vi "estructura basica video tiempo real reconocimiento patrones extraccion de imagen 2.0.vi"() -> ()   [LabVIEW 2024]
uses:
  <vilib>/userDefined/High Color/IMAQdx.ctl
  <vilib>/Python/Open Anaconda Python Session.vi
  <vilib>/vision/driver/NI_Vision_Acquisition_Software.lvlib
  <vilib>/vision/NI_Vision_Development_Module.lvlib
panel:
  in  "Stop All":bool
  in  "Refresh Button":bool
  out "Elapsed Time (s)":dbl
  in  "Array 2":i32[][](array[numeric])
  out "Salida":i32[](array[numeric])
  out "error out":errorcluster
  out "Suma":dbl
  out "min value":u8
  out "max value":u8
  out "Promedio":dbl
  out "IMAGEN PROCESADA":T1(plugin-control)
  in  "Session In":T2="cam1"
  in  "Next":bool
  in  "Parameters (Pattern Matching 1)":T3={"Number of Matches Requested"=3, "Minimum Match Score"=800.0, "Angle Ranges"=[{"Start Angle"=-62.0, "End Angle"=54.0}]}
  out "Image 2":T1(plugin-control)
  out "Image 3":T1(plugin-control)
  in  "Template File Path (Pattern Matching 1)":path=path "C:/Users/cseba/OneDrive/Escritorio/C4.png"
  out "Image 4":T1(plugin-control)
  out "ROI":T4={"Global Rectangle"=[34, 35, 224, 222], "Contours"=[{"Contour Type"=0, "ROI Type"=3, "Points"=[34, 35, 224, 222]}]}
  # "1ER CUADRANTE"
  # "262, 306, 382, 428"
  # "2D0 CUADRANTE"
  # "448, 312, 562, 426"
  # "3ER CUADRANTE"
  # "628, 312, 746, 428"
  # "4TO CUADRANTE"
  # "814, 312, 924, 428"
  # "5TO CUADRANTE"
  # "996, 312, 1110, 424"
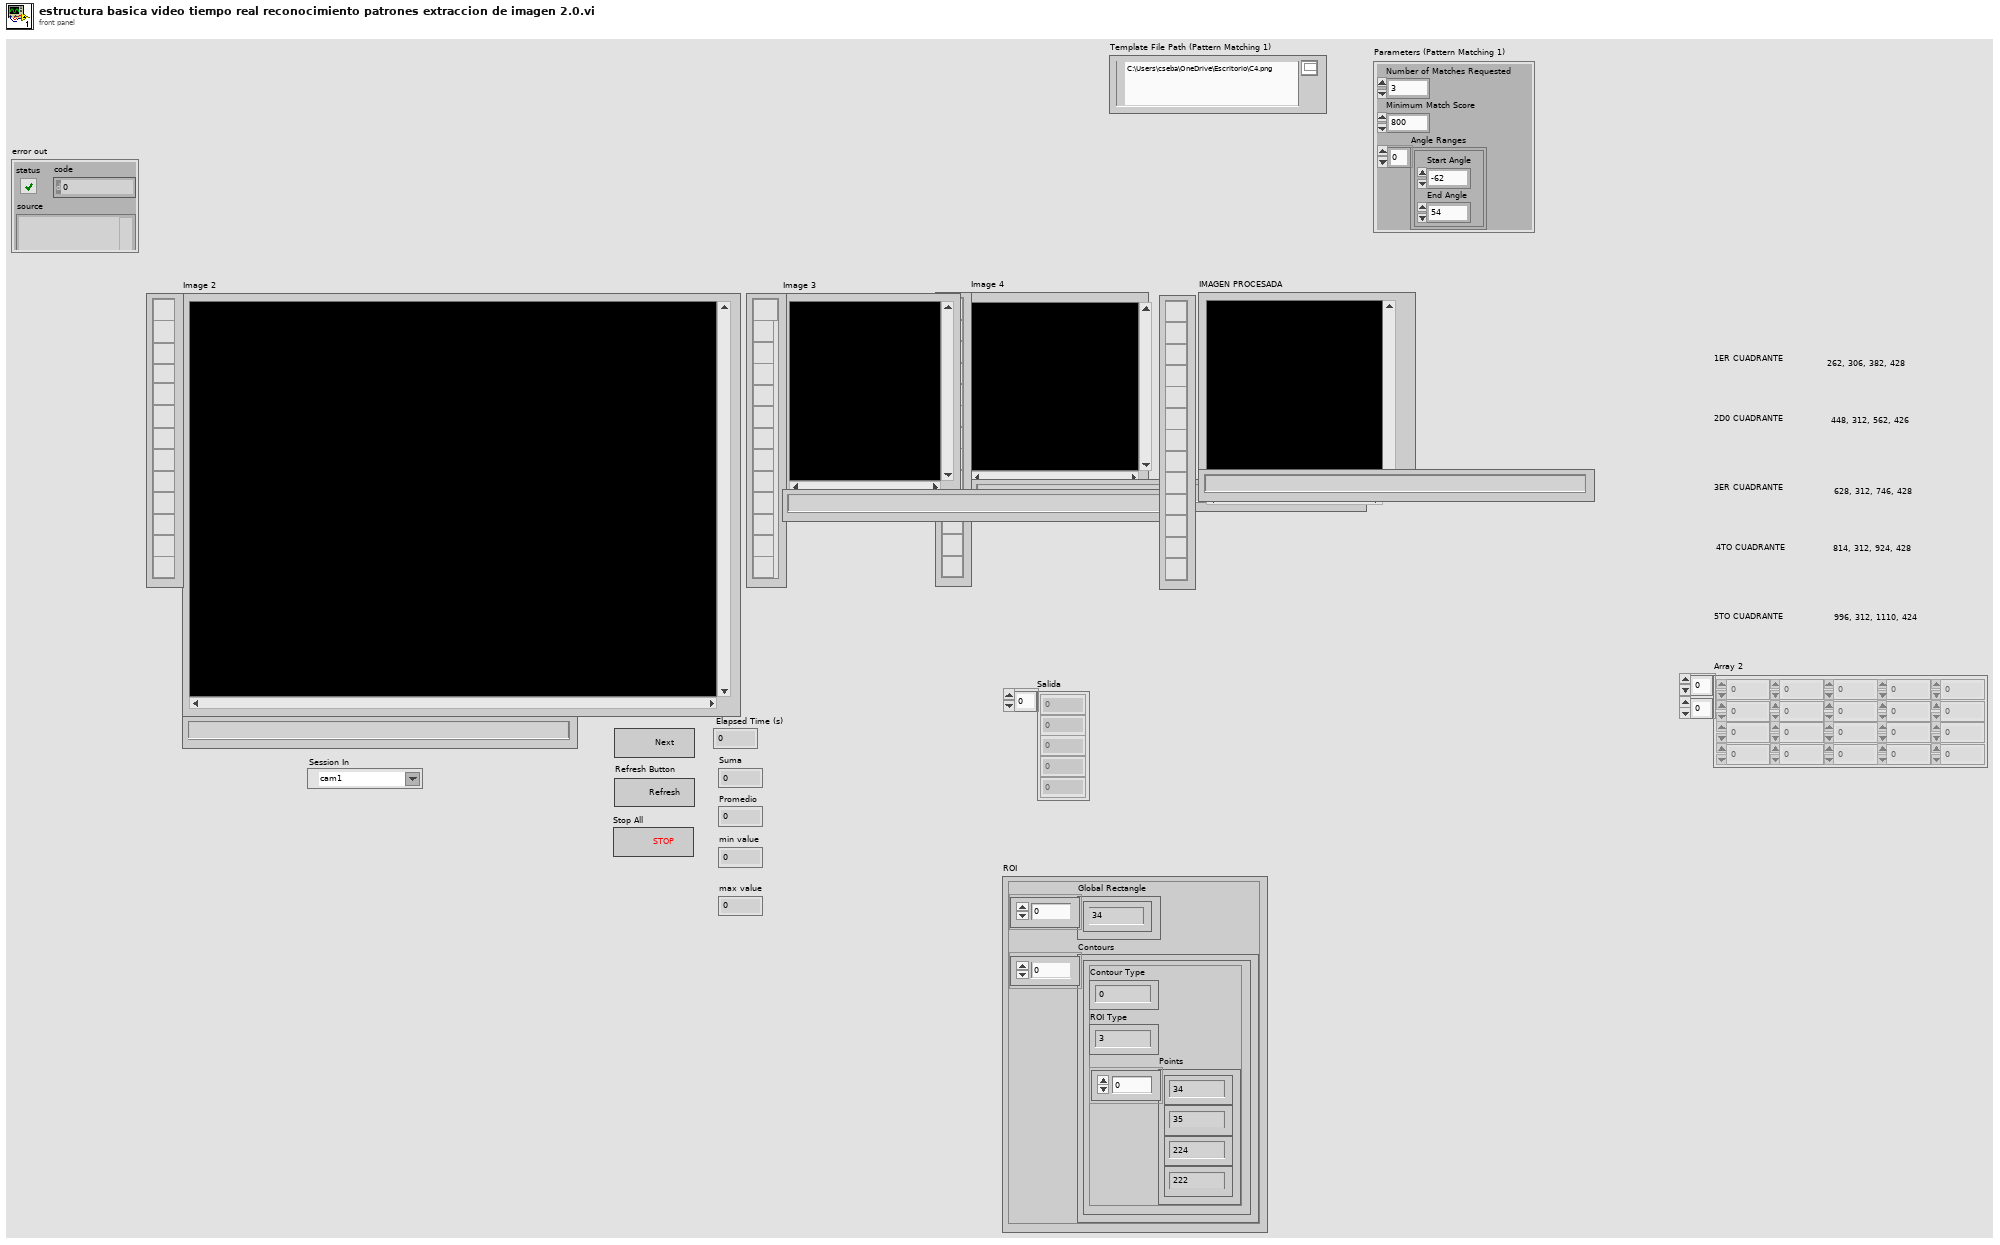
[diagram p1: front panel]
types:
  T1 = typedef "IMAQ Image.ctl" = refnum<image>
  T2 = typedef "IMAQdx.ctl" = refnum<k21>
  T3 = cluster{"Number of Matches Requested":i32, "Minimum Match Score":sgl, "Angle Ranges":cluster{"Start Angle":sgl, "End Angle":sgl}[]}
  T4 = cluster{"Global Rectangle":i32[], "Contours":cluster{"Contour Type":u32, "ROI Type":u32, "Points":i32[]}[]}
  T5 = cluster{"Position":cluster{"x":sgl, "y":sgl}, "Angle":sgl, "Scale":sgl, "Score":sgl, "Bounding Box":cluster{"x":sgl, "y":sgl}[]}[]
  T6 = cluster{"Position":cluster{"x":sgl, "y":sgl}, "Angle":sgl, "Scale":sgl, "Score":sgl, "Bounding Box":cluster{"x":sgl, "y":sgl}[]}
  T7 = cluster{"Contour Type":u32, "ROI Type":u32, "Points":i32[]}[]
  T8 = cluster{"Contour Type":u32, "ROI Type":u32, "Points":i32[]}
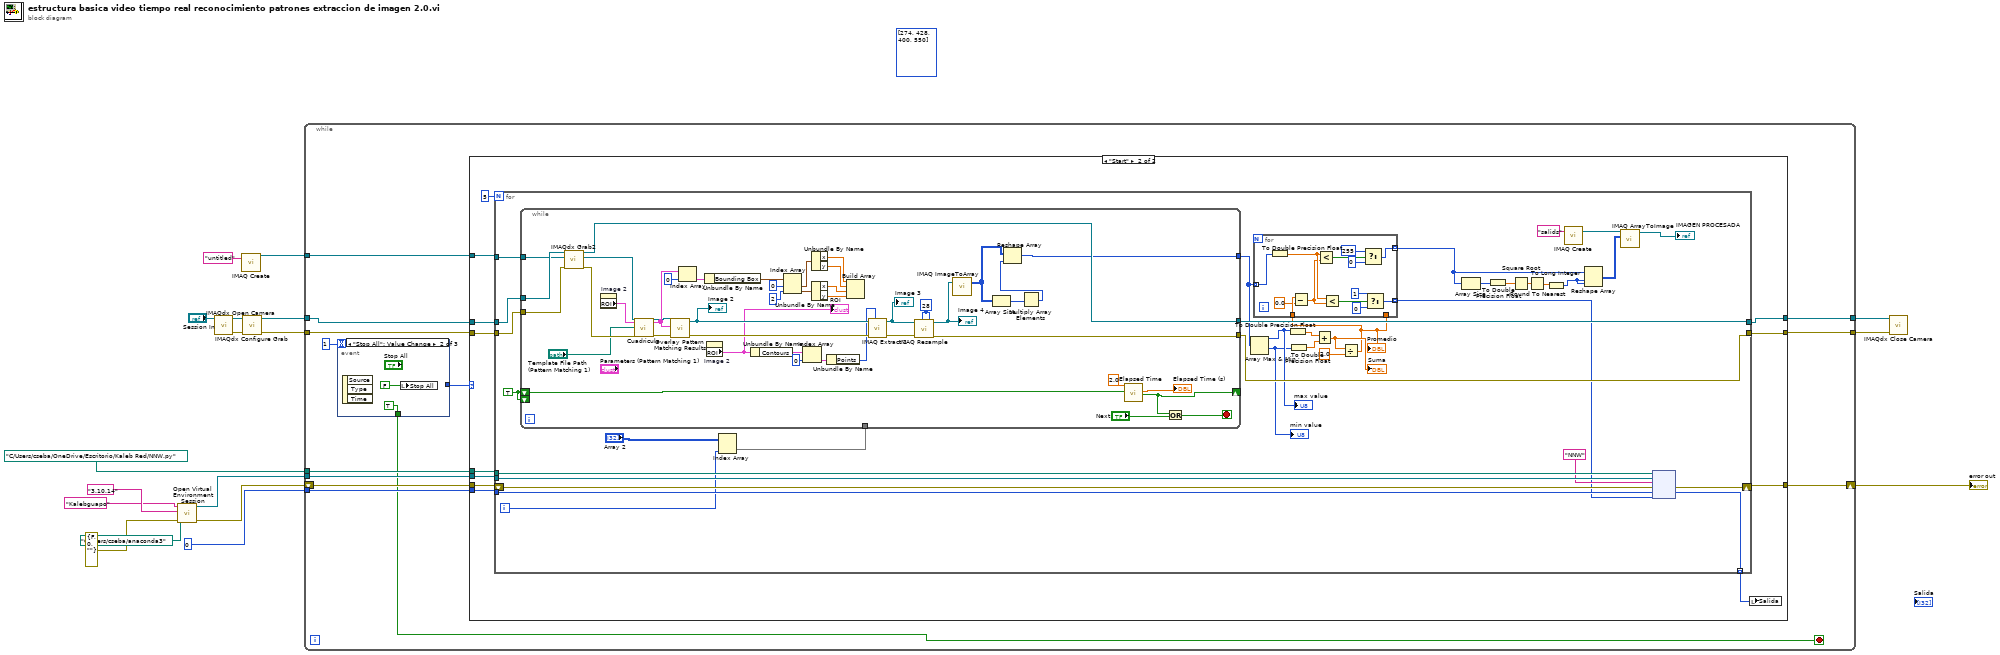
[diagram p0: block diagram]
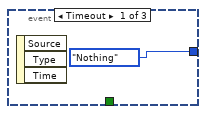
[diagram p2: hidden frame]
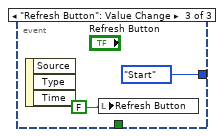
[diagram p3: hidden frame]
diagram:
  (unwired) i32[] [274, 428, 400, 550]
  n1 = call-poly <vilib>:"Open Virtual Environment Session.vi"("error in (no error)"=errorcluster {"status"=FALSE, "code"=0, "source"=""}, "Anaconda path"=path "C:/Users/cseba/anaconda3", "Python version"="3.10.14", "Env name"="Kalebguapo") -> ("error out"=w5:errorcluster, "session out"=w7:refnum<k35>)  [unwired: 6 in]
  n2 = call <vilib>:"IMAQdx Open Camera.vi"("Session In"="Session In") -> ("error out"=w16:errorcluster, "Session Out"=w17:T2)  [unwired: 9 in]
  n3 = call "IMAQ Create"("Image Name"="untitled") -> ("New Image"=w12:T1)  [unwired: 4 in, 1 out]
  n4 = call <vilib>:"IMAQdx Configure Grab.vi"("error in"=w16, "Session In"=w17) -> ("error out"=w13:errorcluster, "Session Out"=w14:T2)  [unwired: 8 in]
  n5 = while {
    tunnel: w12 -> [w29]
    tunnel: w7 -> [w26]
    tunnel: path "C:/Users/cseba/OneDrive/Escritorio/Kaleb Red/NNW.py" ("module path") -> [w25]
    tunnel: 0 ("code 2") -> [w22]
    shift-right: [w23] -> w4
    shift-left: w5 -> [w24]
    tunnel: w14 -> [w31]
    tunnel: [w28] -> w11
    tunnel: w13 -> [w30]
    tunnel: [w27] -> w10
    stop <- w19 stop-if-true
    n6 = event shown="[1] \"Stop All\": Value Change" {
      selector: _ -> [_ _ _]
      dyn-events: _ -> [_ _ _]
      timeout: 1 -> [_ _ _]
      tunnel: [enum16{"Nothing", "Start"}."Nothing" ("Enum") _ enum16{"Nothing", "Start"}."Start" ("Enum")] -> w20
      tunnel: [_ TRUE _] -> w19
      event Timeout {
        n7 = event-data() -> ()  [unwired: 1 in, 3 out]
      }
      event "Stop All": Value Change {
        n8 = event-data() -> ()  [unwired: 1 in, 3 out]
        n9 = local write "Stop All"(FALSE ("Stop All")) -> ()
      }
      event "Refresh Button": Value Change {
        n10 = event-data() -> ()  [unwired: 1 in, 3 out]
        n11 = local write "Refresh Button"(FALSE ("Refresh Button")) -> ()
      }
    }
    n12 = case shown="\"Start\"" w20 {
      tunnel: w31 -> [w39 w51]
      tunnel: w30 -> [w38 w50]
      tunnel: w29 -> [_ w49]
      tunnel: [w39 w48] -> w28
      tunnel: [w38 w47] -> w27
      tunnel: w26 -> [_ w46]
      tunnel: w25 -> [_ w45]
      tunnel: w24 -> [w37 w44]
      tunnel: [w37 w43] -> w23
      tunnel: w22 -> [_ w42]
      frame "Nothing", Default {
      }
      frame "Start" {
        n13 = for {
          N: 5 -> [_]
          tunnel: w49 -> [w84]
          tunnel: w46 -> [w64]
          tunnel: w45 -> [w63]
          tunnel: w42 -> [w59]
          shift-right: [w61] -> w43
          shift-left: w44 -> [w62]
          tunnel: [w56] -> w40 mode=indexing
          tunnel: w51 -> [w86]
          tunnel: [w83] -> w48
          tunnel: w50 -> [w85]
          tunnel: [w82] -> w47
          i -> [w54]
          w52 = TRUE ("Reset")
          n14 = Index Array(array="Array 2", index (col)=w54) -> (element=w53:i32[])  [unwired: 1 in]
          n15 = while {
            tunnel: w86 -> [w143]
            tunnel: w85 -> [w142]
            tunnel: w84 -> [w141]
            tunnel: [w119] -> w83
            tunnel: [w126] -> w82
            tunnel: [w117] -> w81
            tunnel: w53 -> [_]
            shift-right: [w102] -> _
            shift-left: w52 -> [w103]
            shift-left: w52 -> [_]
            stop <- w104 stop-if-true
            w125 = 28
            n16 = call <vilib>:"IMAQdx Grab2.vi"("error in"=w142, "Image In"=w141, "Session In"=w143) -> ("error out"=w110:errorcluster, "Image Out"=w139:T1, "Session Out"=w119:T2)  [unwired: 5 in, 1 out]
            n17 = property on="Image 2" class="ImageControl"() -> ("ROI"=w109:T4)  [unwired: 2 in, 2 out]
            n18 = call "Cuadricula.vi"("Image In"=w139, "ROI Descriptor (Pattern Matching 1)"=w109, "Template File Path (Pattern Matching 1)"="Template File Path (Pattern Matching 1)", "error in"=w110) -> ("Image Out"=w138:T1, "Matches (Pattern Matching 1)"=w114:T5, "error out"=w140:errorcluster)  [unwired: 20 in, 1 out]
            n19 = call "Overlay Pattern Matching Results.vi"("error in"=w140, "Matches"=w114, "Image"=w138) -> ("error out"=w112:errorcluster, "Image Out"=w113:T1)  [unwired: 7 in]
            "Image 2" <- w113
            n20 = Index Array(array=w114, index=0) -> (element=w136:T6)
            n21 = Unbundle By Name(w136) -> ("Bounding Box"=w134:cluster{"x":sgl, "y":sgl}[])
            n22 = property on="Image 2" class="ImageControl"() -> ("ROI"=w108:T4)  [unwired: 2 in, 2 out]
            "ROI" <- w108
            n23 = Unbundle By Name(w108) -> ("Contours"=w124:T7)
            n24 = Index Array(array=w134, index #1=0 ("index"), index #2=2 ("index")) -> (element #1=w132:cluster{"x":sgl, "y":sgl}, element #2=w129:cluster{"x":sgl, "y":sgl})
            n25 = Index Array(array=w124, index=0) -> (element=w122:T8)
            n26 = Unbundle By Name(w132) -> ("x"=w135:sgl, "y"=w131:sgl)
            n27 = Unbundle By Name(w129) -> ("x"=w128:sgl, "y"=w127:sgl)
            n28 = Unbundle By Name(w122) -> ("Points"=w101:i32[])
            n29 = Build Array(w135, w131, w128, w127) -> ()  [unwired: 1 out]
            n30 = call "IMAQ Extract 2"("Optional Rectangle"=w101, "error in (no error)"=w112, "Image Src"=w113) -> ("error out"=w115:errorcluster, "Image Dst Out"=w116:T1)  [unwired: 7 in]
            "Image 3" <- w116
            n31 = call "IMAQ Resample"("X Resolution"=w125, "Y Resolution"=w125, "error in (no error)"=w115, "Image Src"=w116) -> ("error out"=w126:errorcluster, "Image Dst Out"=w121:T1)  [unwired: 6 in]
            "Image 4" <- w121
            n32 = call "IMAQ ImageToArray"("Image"=w121) -> ("Image Pixels (U8)"=w111:u8[][])  [unwired: 3 in, 4 out]
            n33 = Array Size(array=w111) -> (size(s)=w120:i32[])
            n34 = Multiply Array Elements(1:w120) -> (0:w118:i32)
            n35 = Reshape Array(w111, w118) -> (w117:u8[])
            n36 = call "Elapsed Time"("Time Target (s)"=2.0, "Reset"=w103) -> ("Elapsed Time (s)"=→"Elapsed Time (s)":dbl, "Time has Elapsed"=w102:bool)  [unwired: 10 in, 6 out]
            n37 = Or(x=w102, y="Next") -> (x .or. y?=w104:bool)
          }
          n38 = Array Max & Min(array=w81) -> (max value=w68:u8, min value=w67:u8)  [unwired: 2 out]
          "max value" <- w68
          "min value" <- w67
          n39 = To Double Precision Float(number=w68) -> (double precision float=w70:dbl)
          n40 = To Double Precision Float(number=w67) -> (double precision float=w69:dbl)
          n41 = Add(x=w70, y=w69) -> (x+y=w66:dbl)
          "Suma" <- w66
          n42 = Divide(x=w66, y=2.0) -> (x/y=w65:dbl)
          "Promedio" <- w65
          n43 = for {
            tunnel: w81 -> [w99] mode=indexing
            tunnel: w65 -> [w94]
            tunnel: [w95] -> w58 mode=indexing
            tunnel: w65 -> [_]
            tunnel: [w87] -> w57 mode=indexing
            n44 = To Double Precision Float(number=w99) -> (double precision float=w92:dbl)
            n45 = Subtract(x=w94, y=0.0) -> (x-y=w91:dbl)
            n46 = Less?(x=w92, y=w91) -> (x < y?=w98:bool)
            n47 = Less?(x=w92, y=w91) -> (x < y?=w90:bool)
            n48 = Select(t=u8 255, s=w98, f=u8 0) -> (s? t:f=w95:u8)
            n49 = Select(t=u8 1, s=w90, f=u8 0 ("t")) -> (s? t:f=w87:u8)
          }
          n50 = Array Size(array=w58) -> (size(s)=w78:i32)
          n51 = To Double Precision Float(number=w78) -> (double precision float=w77:dbl)
          n52 = Square Root(x=w77) -> (sqrt(x)=w76:dbl)
          n53 = Round To Nearest(number=w76) -> (nearest integer value=w75:dbl)
          n54 = To Long Integer(number=w75) -> (32bit integer=w74:i32)
          n55 = call "IMAQ Create"("Image Name"="salids") -> ("New Image"=w79:T1)  [unwired: 4 in, 1 out]
          n56 = Reshape Array(w58, w74, w74) -> (w72:u8[][])
          n57 = call "IMAQ ArrayToImage"("Image Pixels (U8)"=w72, "Image"=w79) -> ("Image Out"=→"IMAGEN PROCESADA":T1)  [unwired: 8 in, 1 out]
          n58 = node(w64, w63, "NNW" ("function name"), w62, w59, w57) -> (w61:errorcluster, w56:i32)  [unwired: 1 in, 3 out]
        }
        n59 = local write "Salida"(w40) -> ()
      }
    }
  }
  "error out" <- w4
  n60 = call <vilib>:"IMAQdx Close Camera.vi"("error in"=w10, "Session In"=w11) -> ()  [unwired: 9 in, 1 out]
